vi "Alarm Clock 2012 NIVerified.vi"() -> ()   [LabVIEW 2012]
doc: "This is an example can display the time and date and you can also set an alarm. The LED lights when the alarm rings, and you can choose to turn off the alarm clock or 5 minutes snooze."
panel:
  in  "Variabe":bool
  out "error out":errorcluster
  out "Date":string
  in  "x 3":dbl
  in  "Hour":dbl
  in  "Mintues":dbl
  out "Alarm":bool
  in  "Set Alarm":bool
  out "Time":string
  in  "error in":errorcluster caption="error in (no error)"
  # "Overview: This a simple alarm clock that lets displays the time and date. It also lets you\n set an alarm and lights an LED when it rings. It also has a 5 minute snooze.\nRequirements: LabVIEW 2012 (or compatible)\nInstructions:\n1. Run the VI.\n2. Time and Date indicator display the current time and date.\n3. Click Alarm control to set  hour and minutes of alarm."
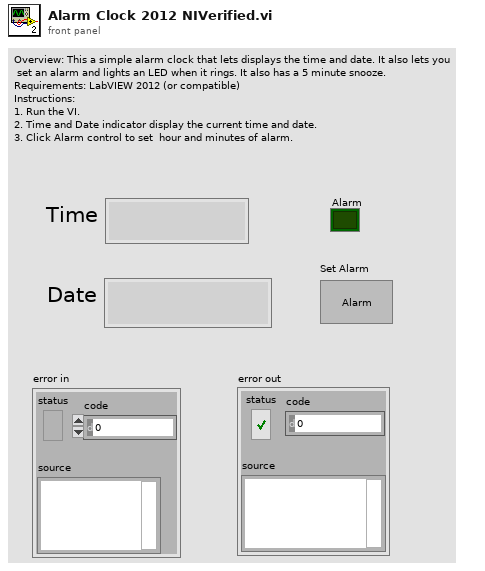
[diagram p1: front panel]
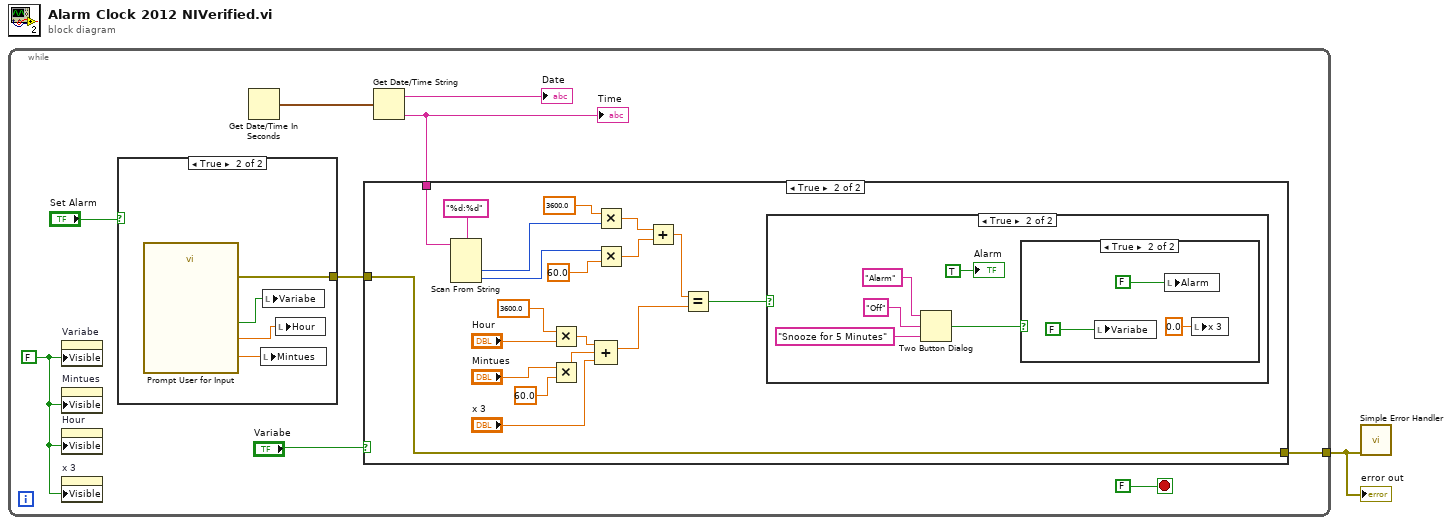
[diagram p0: block diagram]
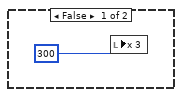
[diagram p4: hidden frame]
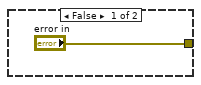
[diagram p5: hidden frame]
diagram:
  n1 = while {
    tunnel: [w4] -> w1
    stop <- FALSE stop-if-true
    w7 = FALSE ("Visible")
    n2 = property on="Variabe" class="Bool (strict)"("Visible"=w7) -> ()  [unwired: 2 in, 2 out]
    n3 = property on="Mintues" class="DigNum (strict)"("Visible"=w7) -> ()  [unwired: 2 in, 2 out]
    n4 = property on="Hour" class="DigNum (strict)"("Visible"=w7) -> ()  [unwired: 2 in, 2 out]
    n5 = property on="x 3" class="DigNum (strict)"("Visible"=w7) -> ()  [unwired: 2 in, 2 out]
    n6 = case shown="True" "Set Alarm" {
      tunnel: ["error in" w41] -> w5
      frame False {
      }
      frame True {
        n7 = call "Prompt User for Input"() -> ("Minute"=w42:dbl, "Hour"=w43:dbl, "OK"=w44:bool, "error out"=w41:errorcluster)  [unwired: 16 in]
        n8 = local write "Mintues"(w42) -> ()
        n9 = local write "Variabe"(w44) -> ()
        n10 = local write "Hour"(w43) -> ()
      }
    }
    n11 = Get Date/Time In Seconds() -> (seconds since 1Jan1904=w8:timestamp)
    n12 = Get Date/Time String(seconds (now)=w8) -> (date string=→"Date":string, time string=w3:string)  [unwired: 2 in]
    "Time" <- w3
    n13 = case shown="True" "Variabe" {
      tunnel: w3 -> [_ w19]
      tunnel: w5 -> [w11 w15]
      tunnel: [w11 w15] -> w4
      frame False {
      }
      frame True {
        n14 = Scan From String(format string="%d:%d", input string=w19) -> (output 1=w18:i32, output 2=w17:i32)  [unwired: 4 in, 3 out]
        n15 = Multiply(x=3600.0, y="Hour") -> (x*y=w28:dbl)
        n16 = Multiply(x="Mintues", y=60.0) -> (x*y=w27:dbl)
        n17 = Compound Arithmetic op=ADD(w28, w27, "x 3") -> (w25:dbl)
        n18 = Multiply(x=3600.0, y=w18) -> (x*y=w22:dbl)
        n19 = Multiply(x=w17, y=60.0) -> (x*y=w21:dbl)
        n20 = Add(x=w22, y=w21) -> (x+y=w20:dbl)
        n21 = Equal?(x=w20, y=w25) -> (x = y?=w12:bool)
        n22 = case shown="True" w12 {
          frame False {
          }
          frame True {
            n23 = Two Button Dialog(message="Alarm", 1:"Snooze for 5 Minutes" ("F button name (\"Cancel\")"), 2:"Off" ("T button name (\"OK\")")) -> (T button?=w32:bool)
            n24 = case shown="True" w32 {
              frame False {
                n25 = local write "x 3"(300) -> ()
              }
              frame True {
                n26 = local write "Variabe"(FALSE ("variabe")) -> ()
                n27 = local write "Alarm"(FALSE ("Alarm")) -> ()
                n28 = local write "x 3"(0.0 ("x 3")) -> ()
              }
            }
            "Alarm" <- TRUE ("Boolean")
          }
        }
      }
    }
  }
  "error out" <- w1
  n29 = call <vilib>:"Simple Error Handler.vi"("error in (no error)"=w1) -> ()  [unwired: 4 in, 5 out]
